vi "getLocalRepoId.vi"(8 "error in (no error)":errorcluster, 11 "svnHandler in":refnum<class "svnHandler.lvclass">) -> (0 "error out":errorcluster, 3 "svnHandler out":refnum<class "svnHandler.lvclass">)   [LabVIEW 2013, in "svnHandler.lvclass"]
uses:
  svnHandler.lvclass
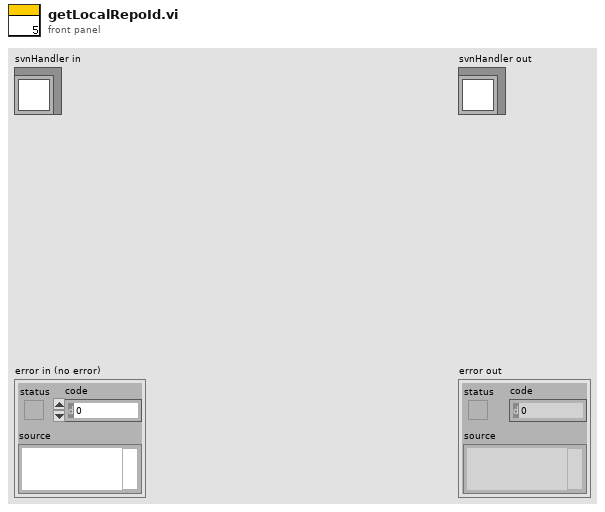
[diagram p1: front panel]
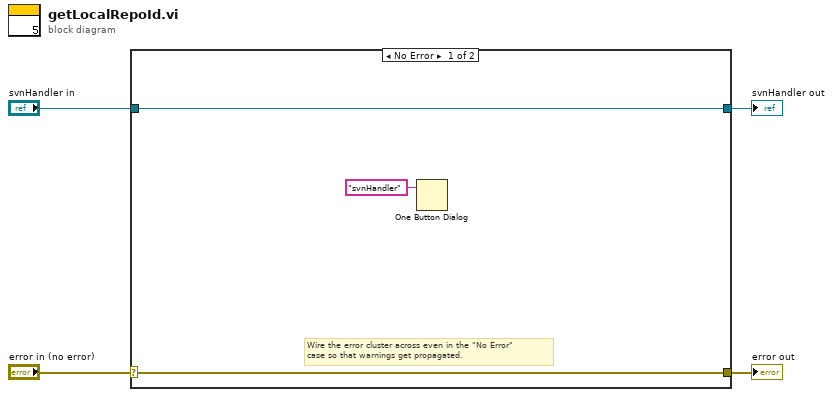
[diagram p0: block diagram]
diagram:
  n1 = case shown="No Error" "error in (no error)" {
    selector: "error in (no error)" -> [w6 w9]
    tunnel: [w6 w9] -> w3
    tunnel: [w7 w8] -> w1
    tunnel: "svnHandler in" -> [w7 w8]
    frame No Error {
      # "Wire the error cluster across even in the \"No Error\"\ncase so that warnings get propagated."
      n2 = One Button Dialog(message="svnHandler") -> ()  [unwired: 1 in, 1 out]
    }
    frame Error {
    }
  }
  "error out" <- w3
  "svnHandler out" <- w1
